vi "Write RP Instrument.lvclass.vi"(8 "error in (no error)":errorcluster, 10 "RP Instrument.lvclass":refnum<class "RP Instrument.lvclass">, 11 "Red Pitaya Digitizer in":refnum<class "Red Pitaya Recorder.lvclass">) -> (0 "error out":errorcluster, 3 "Red Pitaya Digitizer out":refnum<class "Red Pitaya Recorder.lvclass">)   [LabVIEW 2015, in "Red Pitaya Recorder.lvclass"]
uses:
  Red Pitaya Recorder.lvclass
  NHMFL_Core/Libraries/Red Pitaya/RP Core/RP Instrument/RP Instrument.lvclass
  Red Pitaya Recorder.lvclass/Red Pitaya Recorder.ctl
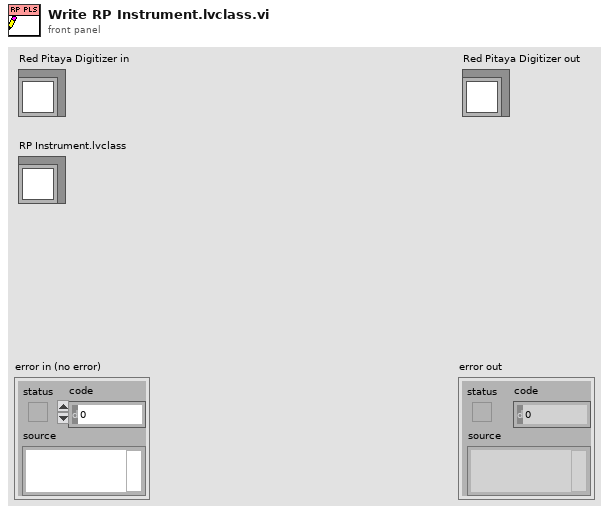
[diagram p1: front panel]
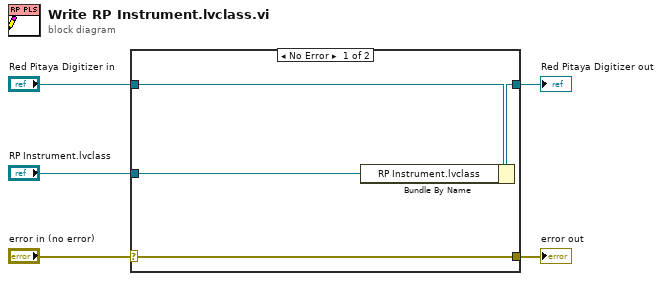
[diagram p0: block diagram]
diagram:
  n1 = case shown="No Error" "error in (no error)" {
    selector: "error in (no error)" -> [w9 w10]
    tunnel: [w9 w10] -> w4
    tunnel: [w7 w11] -> w2
    tunnel: "Red Pitaya Digitizer in" -> [w8 w11]
    tunnel: "RP Instrument.lvclass" -> [w6 _]
    frame No Error {
      n2 = Bundle By Name(cluster=w8, "RP Instrument.lvclass"=w6) -> (w7:refnum<class "Red Pitaya Recorder.lvclass">)
    }
    frame Error {
    }
  }
  "error out" <- w4
  "Red Pitaya Digitizer out" <- w2
